vi "HandleServers.vi"(8 "error in (no error)":errorcluster, 11 "S4ACS_GUI in":refnum<class "S4ACS_GUI.lvclass">) -> (0 "error out":errorcluster, 3 "S4ACS_GUI out":refnum<class "S4ACS_GUI.lvclass">)   [LabVIEW 2018, in "S4ACS_GUI.lvclass"]
uses:
  S4ACS_GUI.lvclass
  S4ACS_GUI.lvclass/S4ACS_GUI.ctl
  Acquisition/Acquisition.lvclass
  SyncBox/Sync Box.lvclass
  Instrument/Instrument.lvclass
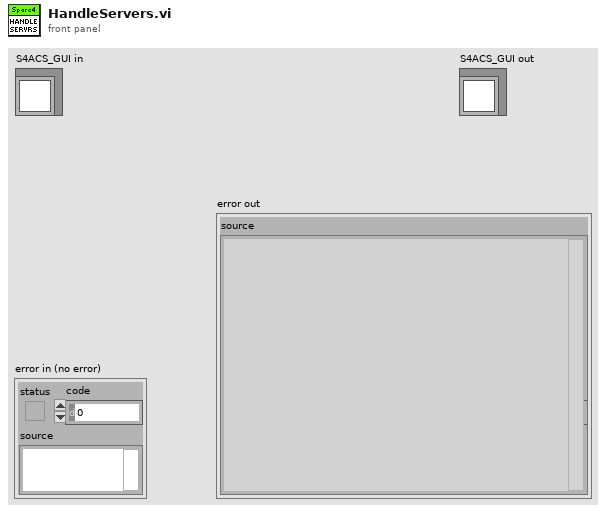
[diagram p1: front panel]
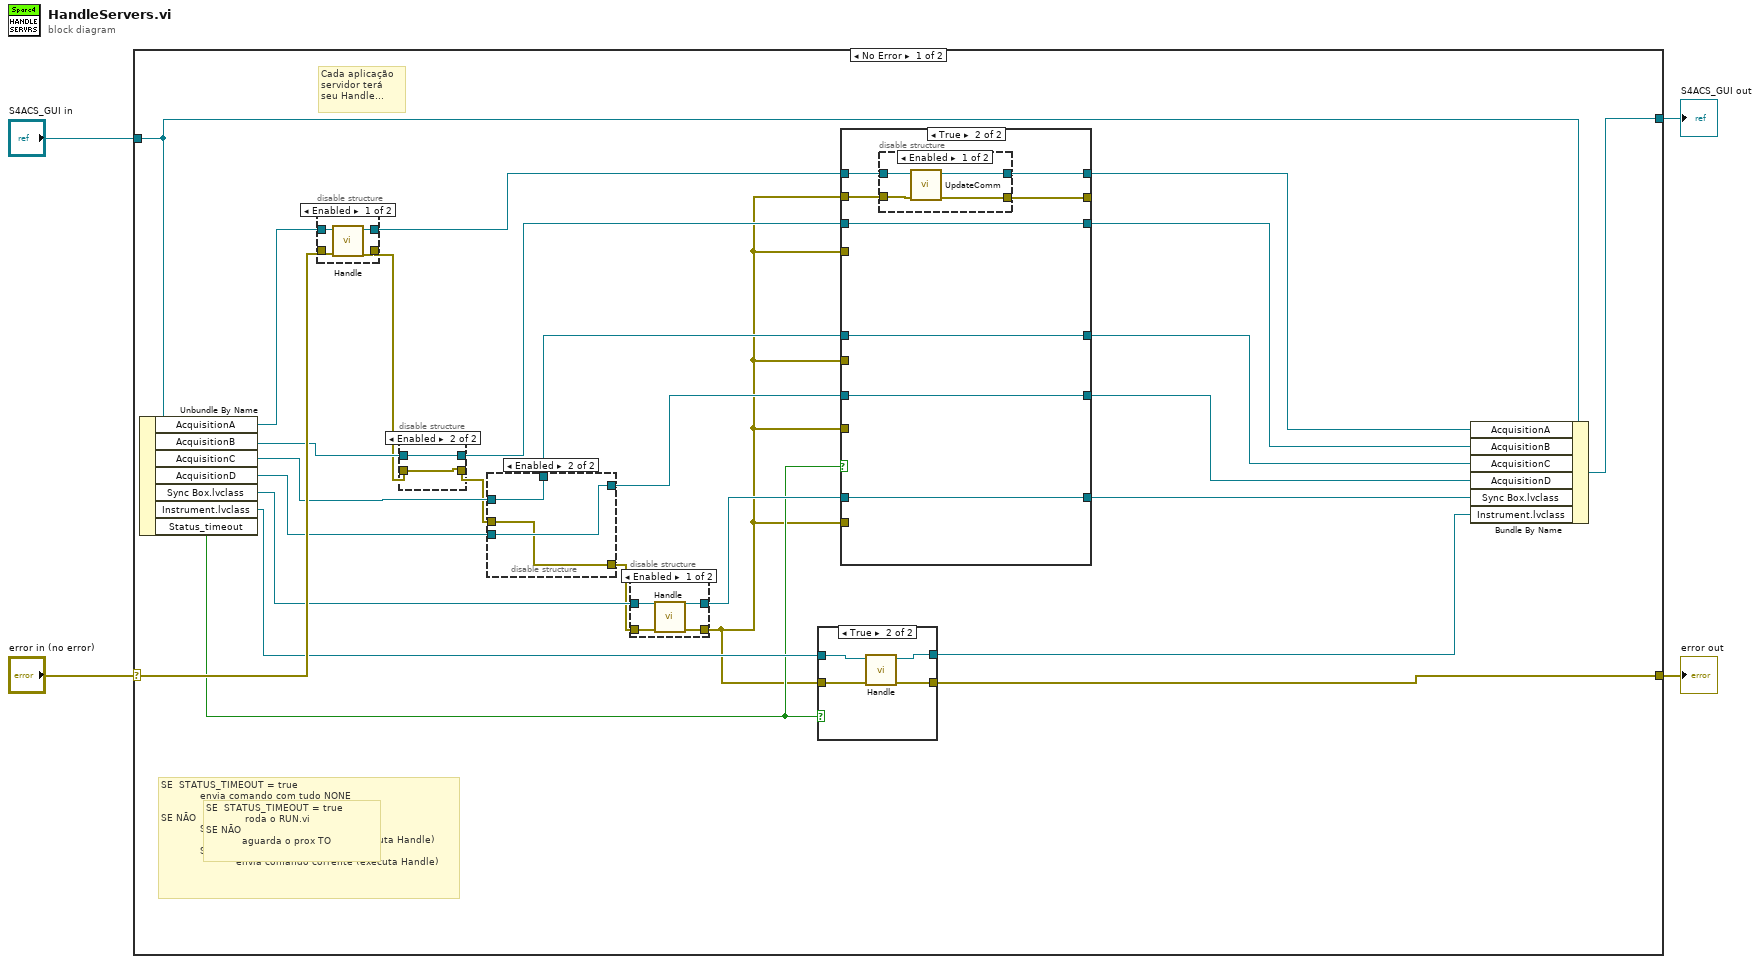
[diagram p0: block diagram]
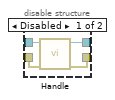
[diagram p4: hidden frame]
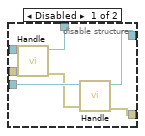
[diagram p5: hidden frame]
diagram:
  n1 = case shown="No Error" "error in (no error)" {
    selector: "error in (no error)" -> [w29 w86]
    tunnel: [w20 w86] -> w3
    tunnel: [w26 w85] -> w1
    tunnel: "S4ACS_GUI in" -> [w27 w85]
    frame No Error {
      # "SE  STATUS_TIMEOUT = true\n             roda o RUN.vi\nSE NÃO\n            aguarda o prox TO"
      # "SE  STATUS_TIMEOUT = true\n             envia comando com tudo NONE\n              e não executa Handle\nSE NÃO\n             SE TODOS ESTADOS = 0\n                        Não envia comando (nao executa Handle)\n             SE NAO\n                         envia comando corrente (executa Handle)"
      # "Cada aplicação \nservidor terá \nseu Handle..."
      n2 = Unbundle By Name(w27) -> ("AcquisitionA"=w30:refnum<class "Acquisition.lvclass">, "AcquisitionB"=w28:refnum<class "Acquisition.lvclass">, "AcquisitionC"=w23:refnum<class "Acquisition.lvclass">, "AcquisitionD"=w22:refnum<class "Acquisition.lvclass">, "Sync Box.lvclass"=w25:refnum<class "Sync Box.lvclass">, "Instrument.lvclass"=w19:refnum<class "Instrument.lvclass">, "Status_timeout"=w10:bool)
      n3 = disable-structure shown="Enabled" {
        disable-tunnel: w30 -> [w70 w72]
        disable-tunnel: w29 -> [w69 w71]
        disable-tunnel: [w68 w72] -> w11
        disable-tunnel: [w67 w71] -> w21
        frame Enabled {
          n4 = call-dynamic "Handle.vi"("error in (no error)"=w69, "Acquisition in"=w70) -> ("error out"=w67:errorcluster, "Acquisition out"=w68:refnum<class "Acquisition.lvclass">)  [unwired: 8 in]
        }
        frame Disabled {
        }
      }
      n5 = disable-structure shown="Enabled" {
        disable-tunnel: w28 -> [w54 w55]
        disable-tunnel: [w53 w55] -> w12
        disable-tunnel: w21 -> [w52 w56]
        disable-tunnel: [w51 w56] -> w18
        frame Disabled {
          n6 = call-dynamic "Handle.vi"("error in (no error)"=w52, "Acquisition in"=w54) -> ("error out"=w51:errorcluster, "Acquisition out"=w53:refnum<class "Acquisition.lvclass">)  [unwired: 8 in]
        }
        frame Enabled {
        }
      }
      n7 = disable-structure shown="Enabled" {
        disable-tunnel: [w63 w64] -> w24
        disable-tunnel: w23 -> [w62 w66]
        disable-tunnel: w22 -> [w61 w65]
        disable-tunnel: [w60 w65] -> w14
        disable-tunnel: [w59 w66] -> w13
        disable-tunnel: w18 -> [w58 w64]
        frame Disabled {
          n8 = call-dynamic "Handle.vi"("error in (no error)"=w58, "Acquisition in"=w62) -> ("error out"=w57:errorcluster, "Acquisition out"=w59:refnum<class "Acquisition.lvclass">)  [unwired: 8 in]
          n9 = call-dynamic "Handle.vi"("error in (no error)"=w57, "Acquisition in"=w61) -> ("error out"=w63:errorcluster, "Acquisition out"=w60:refnum<class "Acquisition.lvclass">)  [unwired: 8 in]
        }
        frame Enabled {
        }
      }
      n10 = disable-structure shown="Enabled" {
        disable-tunnel: [w82 w83] -> w9
        disable-tunnel: w25 -> [w81 w84]
        disable-tunnel: [w80 w84] -> w16
        disable-tunnel: w24 -> [w79 w83]
        frame Enabled {
          n11 = call-dynamic "Handle.vi"("error in (no error)"=w79, "Sync Box in"=w81) -> ("error out"=w82:errorcluster, "Sync Box out"=w80:refnum<class "Sync Box.lvclass">)  [unwired: 8 in]
        }
        frame Disabled {
        }
      }
      n12 = case shown="True" w10 {
        tunnel: [w74 w78] -> w17
        tunnel: [w73 w77] -> w20
        tunnel: w19 -> [w74 w76]
        tunnel: w9 -> [w73 w75]
        frame False {
        }
        frame True {
          n13 = call-dynamic "Handle.vi"("error in (no error)"=w75, "Instrument in"=w76) -> ("error out"=w77:errorcluster, "Instrument out"=w78:refnum<class "Instrument.lvclass">)  [unwired: 8 in]
        }
      }
      n14 = case shown="True" w10 {
        tunnel: w16 -> [w32 w44]
        tunnel: [w32 w44] -> w15
        tunnel: w14 -> [w33 w37]
        tunnel: w13 -> [w34 w38]
        tunnel: w12 -> [w35 w39]
        tunnel: w11 -> [w36 w43]
        tunnel: w9 -> [w31 w42]
        tunnel: w9 -> [_ _]
        tunnel: w9 -> [_ _]
        tunnel: w9 -> [_ _]
        tunnel: w9 -> [_ _]
        tunnel: [w36 w41] -> w8
        tunnel: [w35 w39] -> w7
        tunnel: [w34 w38] -> w6
        tunnel: [w33 w37] -> w5
        tunnel: [w31 w40] -> _
        frame False {
        }
        frame True {
          n15 = disable-structure shown="Enabled" {
            disable-tunnel: w43 -> [w48 w50]
            disable-tunnel: w42 -> [w47 w49]
            disable-tunnel: [w46 w50] -> w41
            disable-tunnel: [w45 w49] -> w40
            frame Enabled {
              n16 = call-dynamic "UpdateComm.vi"("error in (no error)"=w47, "Acquisition in"=w48) -> ("error out"=w45:errorcluster, "Acquisition out"=w46:refnum<class "Acquisition.lvclass">)  [unwired: 8 in]
            }
            frame Disabled {
            }
          }
        }
      }
      n17 = Bundle By Name(cluster=w27, "AcquisitionA"=w8, "AcquisitionB"=w7, "AcquisitionC"=w6, "AcquisitionD"=w5, "Sync Box.lvclass"=w15, "Instrument.lvclass"=w17) -> (w26:refnum<class "S4ACS_GUI.lvclass">)
    }
    frame Error {
    }
  }
  "error out" <- w3
  "S4ACS_GUI out" <- w1
